vi "_063.vi"() -> ()   [LabVIEW 2024]
panel:
  out "O/p":string[](array[string])
  in  "I/p":string[](array[string])
  # "Remove Duplicate Alphabets :"
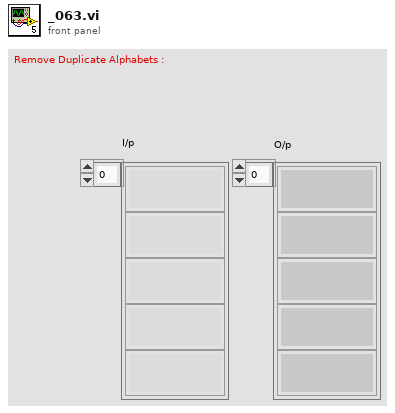
[diagram p1: front panel]
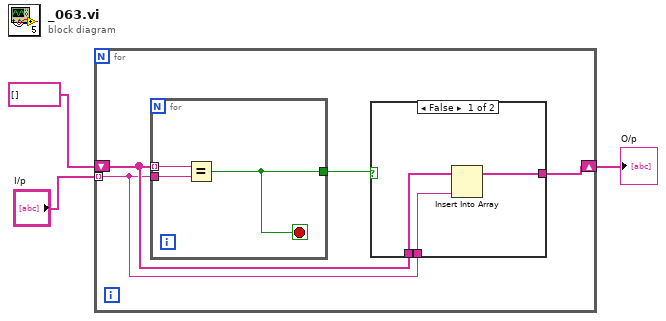
[diagram p0: block diagram]
diagram:
  n1 = for {
    tunnel: "I/p" -> [w5] mode=indexing
    shift-right: [w4] -> w1
    shift-left: string[] [] -> [w6]
    n2 = for {
      tunnel: w6 -> [w14] mode=indexing
      tunnel: w5 -> [w13]
      tunnel: [w12] -> w7
      stop <- w12 stop-if-true
      n3 = Equal?(x=w14, y=w13) -> (x = y?=w12:bool)
    }
    n4 = case shown="False" w7 {
      tunnel: [w10 w11] -> w4
      tunnel: w6 -> [w8 w11]
      tunnel: w5 -> [w9 _]
      frame False {
        n5 = Insert Into Array "Insert Into Array"(array=w8, new element=w9) -> (w10:string[])  [unwired: 1 in]
      }
      frame True {
      }
    }
  }
  "O/p" <- w1
